vi "Extended Periodic 2-Exp Fit Parameters.vi"(8 "Error In":errorcluster, 9 "Laser Period":dbl, 10 "Selected Decay Fit Parameter Array":T1[](array[typedef]), 11 "Decay Fit Parameters":dbl[](array[numeric])) -> (0 "Error Out":errorcluster, 3 "Extended Decay Fit Parameters":dbl[](array[numeric]))   [LabVIEW 2021, in "Fits.lvlib"]
uses:
  Fits.lvlib
  IRF(X)PSED/Decay Fit Parameters & Derived Quantities List.ctl
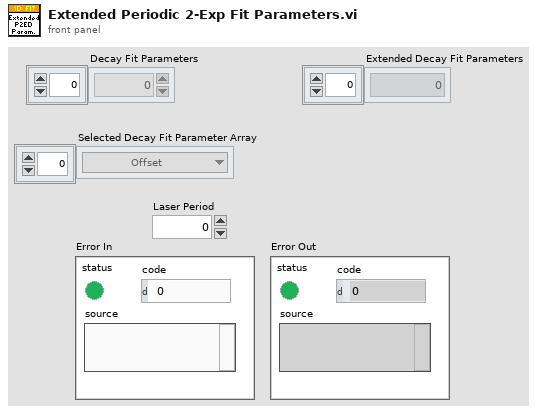
[diagram p1: front panel]
types:
  T1 = typedef "Fits.lvlib/Decay Fit Parameters & Derived Quantities List.ctl" = enum16{"Offset", "Baseline", "A_1", "tau_1", "A_2", "tau_2", "<tau>_1", "f1_1", "f2_1", "<tau>_2", "f1_2", "f2_2", "-", "R^2", "Chi^2"}
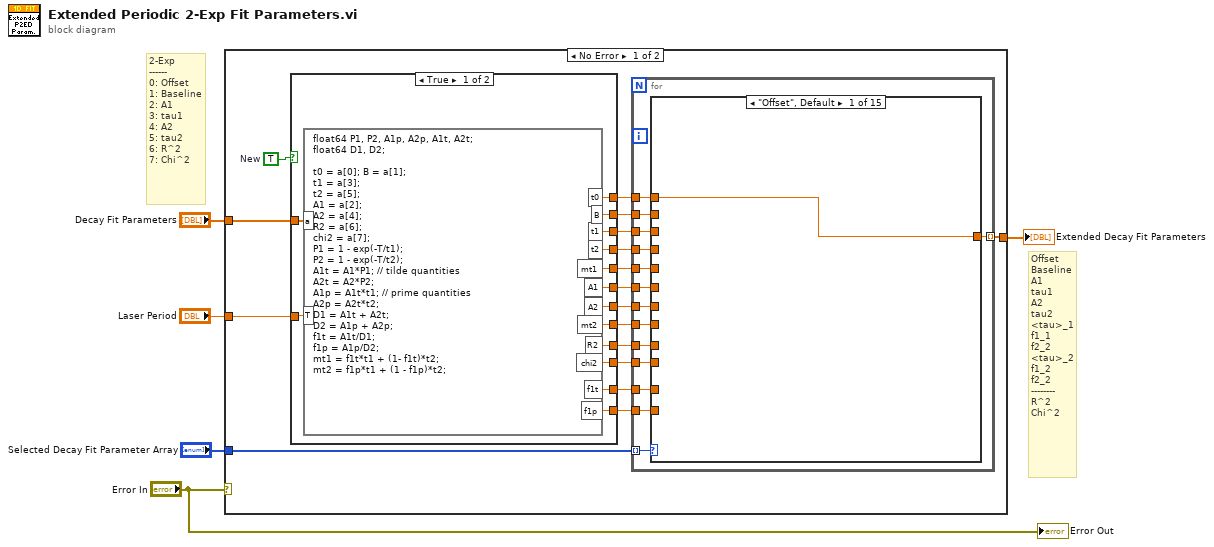
[diagram p0: block diagram]
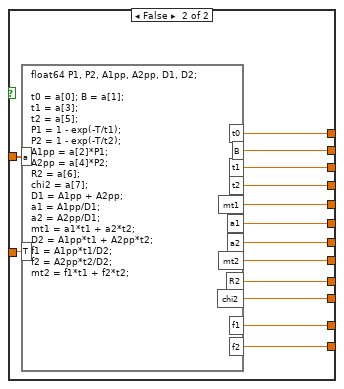
[diagram p2: hidden frame]
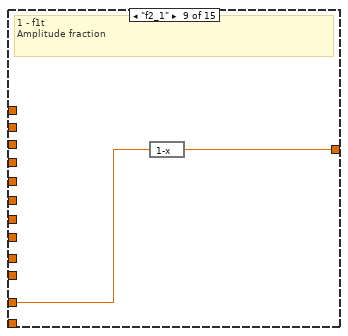
[diagram p10: hidden frame]
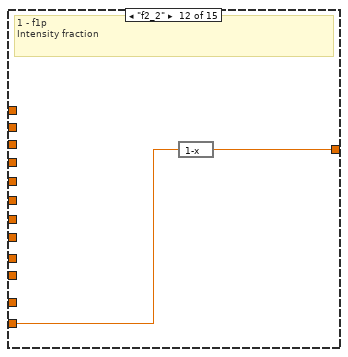
[diagram p13: hidden frame]
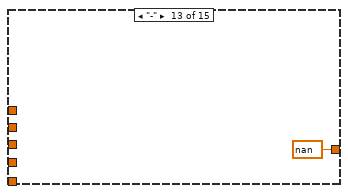
[diagram p14: hidden frame]
diagram:
  # "Offset\nBaseline\nA1\ntau1\nA2\ntau2\n<tau>_1\nf1_1\nf2_2\n<tau>_2\nf1_2\nf2_2\n--------\nR^2\nChi^2"
  # "2-Exp\n------\n0: Offset\n1: Baseline\n2: A1\n3: tau1\n4: A2\n5: tau2\n6: R^2\n7: Chi^2"
  n1 = case shown="No Error" "Error In" {
    tunnel: "Laser Period" -> [w9 _]
    tunnel: "Decay Fit Parameters" -> [w8 _]
    tunnel: "Selected Decay Fit Parameter Array" -> [w7 _]
    tunnel: [w6 _] -> w2
    frame No Error {
      w22 = TRUE  # New
      n2 = case shown="True" w22 {
        tunnel: w8 -> [w36 w50]
        tunnel: w9 -> [w35 w49]
        tunnel: [w34 w48] -> w10
        tunnel: [w33 w47] -> w11
        tunnel: [w32 w46] -> w12
        tunnel: [w31 w45] -> w13
        tunnel: [w30 w44] -> w14
        tunnel: [w29 w43] -> w15
        tunnel: [w28 w42] -> w16
        tunnel: [w27 w41] -> w17
        tunnel: [w26 w40] -> w18
        tunnel: [w25 w39] -> w19
        tunnel: [w24 w38] -> w20
        tunnel: [w23 w37] -> w21
        frame True {
          n3 = formula code="float64 P1, P2, A1p, A2p, A1t, A2t;\nfloat64 D1, D2;\n\nt0 = a[0]; B = a[1];\nt1 = a[3];\nt2 = a[5];\nA1 = a[2];\nA2 = a[4];\nR2 = a[6];\nchi2 = a[7];\nP1 = 1 - exp(-T/t1);\nP2 = 1 - exp(-T/t2);\nA1t = A1*P1; // tilde quantities\nA2t = A2*P2;\nA1p = A1t*t1; // prime quantities\nA2p = A2t*t2;\nD1 = A1t + A2t;\nD2 = A1p + A2p;\nf1t = A1t/D1;\nf1p = A1p/D2;\nmt1 = f1t*t1 + (1- f1t)*t2;\nmt2 = f1p*t1 + (1 - f1p)*t2;"("a"=w36, "T"=w35) -> ("t1"=w30:dbl, "t2"=w29:dbl, "t0"=w34:dbl, "R2"=w33:dbl, "chi2"=w32:dbl, "B"=w31:dbl, "mt1"=w28:dbl, "A1"=w27:dbl, "A2"=w26:dbl, "mt2"=w25:dbl, "f1t"=w24:dbl, "f1p"=w23:dbl)
        }
        frame False {
          n4 = formula code="float64 P1, P2, A1pp, A2pp, D1, D2;\n\nt0 = a[0]; B = a[1];\nt1 = a[3];\nt2 = a[5];\nP1 = 1 - exp(-T/t1);\nP2 = 1 - exp(-T/t2);\nA1pp = a[2]*P1;\nA2pp = a[4]*P2;\nR2 = a[6];\nchi2 = a[7];\nD1 = A1pp + A2pp;\na1 = A1pp/D1;\na2 = A2pp/D1;\nmt1 = a1*t1 + a2*t2;\nD2 = A1pp*t1 + A2pp*t2;\nf1 = A1pp*t1/D2;\nf2 = A2pp*t2/D2;\nmt2 = f1*t1 + f2*t2;"("a"=w50, "T"=w49) -> ("t1"=w44:dbl, "t2"=w43:dbl, "t0"=w48:dbl, "R2"=w47:dbl, "chi2"=w46:dbl, "B"=w45:dbl, "mt1"=w42:dbl, "a1"=w41:dbl, "a2"=w40:dbl, "mt2"=w39:dbl, "f1"=w38:dbl, "f2"=w37:dbl)
        }
      }
      n5 = for {
        tunnel: [w64] -> w6 mode=indexing
        tunnel: w7 -> [w63] mode=indexing
        tunnel: w10 -> [w62]
        tunnel: w11 -> [w61]
        tunnel: w12 -> [w60]
        tunnel: w13 -> [w59]
        tunnel: w14 -> [w58]
        tunnel: w15 -> [w57]
        tunnel: w16 -> [w56]
        tunnel: w17 -> [w55]
        tunnel: w18 -> [w54]
        tunnel: w19 -> [w53]
        tunnel: w20 -> [w52]
        tunnel: w21 -> [w51]
        n6 = case shown="\"Offset\", Default" w63 {
          tunnel: [w65 w66 w67 w68 w69 w70 w71 w72 w73 w75 w76 w77 nan ("chi2") w80 w81] -> w64
          tunnel: w62 -> [w65 _ _ _ _ _ _ _ _ _ _ _ _ _ _]
          tunnel: w61 -> [_ _ _ _ _ _ _ _ _ _ _ _ _ w80 _]
          tunnel: w60 -> [_ _ _ _ _ _ _ _ _ _ _ _ _ _ w81]
          tunnel: w59 -> [_ w66 _ _ _ _ _ _ _ _ _ _ _ _ _]
          tunnel: w58 -> [_ _ _ w68 _ _ _ _ _ _ _ _ _ _ _]
          tunnel: w57 -> [_ _ _ _ _ w70 _ _ _ _ _ _ _ _ _]
          tunnel: w56 -> [_ _ _ _ _ _ w71 _ _ _ _ _ _ _ _]
          tunnel: w55 -> [_ _ w67 _ _ _ _ _ _ _ _ _ _ _ _]
          tunnel: w54 -> [_ _ _ _ w69 _ _ _ _ _ _ _ _ _ _]
          tunnel: w53 -> [_ _ _ _ _ _ _ _ _ w75 _ _ _ _ _]
          tunnel: w52 -> [_ _ _ _ _ _ _ w72 w74 _ _ _ _ _ _]
          tunnel: w51 -> [_ _ _ _ _ _ _ _ _ _ w76 w78 _ _ _]
          frame "Offset", Default {
          }
          frame "Baseline" {
          }
          frame "A_1" {
          }
          frame "tau_1" {
          }
          frame "A_2" {
          }
          frame "tau_2" {
          }
          frame "<tau>_1" {
            # "f1t*t1 +f2t*t2: tilde quantities\nAmplitude-weighted average lifetime"
          }
          frame "f1_1" {
            # "f1t\nAmplitude fraction"
          }
          frame "f2_1" {
            # "1 - f1t\nAmplitude fraction"
            n7 = expression code="1-x"(w74) -> (w73:dbl)
          }
          frame "<tau>_2" {
            # "f1p*t1 + f2p*t2: prime quantities\nIntensity-weighted average lifetime"
          }
          frame "f1_2" {
            # "f1p\nIntensity fraction"
          }
          frame "f2_2" {
            # "1 - f1p\nIntensity fraction"
            n8 = expression code="1-x"(w78) -> (w77:dbl)
          }
          frame "-" {
          }
          frame "R^2" {
          }
          frame "Chi^2" {
          }
        }
      }
    }
    frame Error {
    }
  }
  "Extended Decay Fit Parameters" <- w2
  "Error Out" <- "Error In"
